vi "JTAG Commit.vi"(8 "error in (no error)":errorcluster) -> (0 "error out":errorcluster)   [LabVIEW 2010]
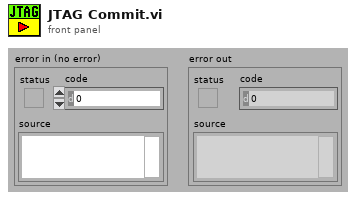
[diagram p1: front panel]
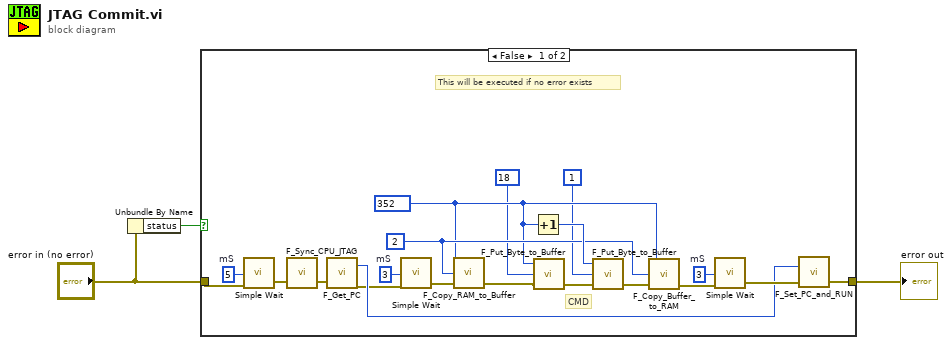
[diagram p0: block diagram]
diagram:
  n1 = Unbundle By Name("error in (no error)") -> ("status"=w2:bool)
  n2 = case shown="False" w2 {
    tunnel: [w10 w24] -> w3
    tunnel: "error in (no error)" -> [w4 w24]
    frame False {
      w6 = u32 5  # mS
      w19 = u32 3  # mS
      w20 = u32 3  # mS
      w16 = u16 2
      w9 = u16 352
      # "CMD"
      # "This will be executed if no error exists"
      n3 = call "Simple Wait.vi"("mS"=w6, "error in"=w4) -> ("error out"=w5:errorcluster)  [unwired: 12 in, 1 out]
      n4 = call "F_Sync_CPU_JTAG.vi"("error in (no error)"=w5) -> ("error out"=w13:errorcluster)  [unwired: 1 in, 1 out]
      n5 = call "F_Get_PC.vi"("error in (no error)"=w13) -> ("error out"=w11:errorcluster, "Program Counter"=w12:u16)  [unwired: 1 in]
      n6 = call "Simple Wait.vi"("mS"=w20, "error in"=w11) -> ("error out"=w17:errorcluster)  [unwired: 12 in, 1 out]
      n7 = call "F_Copy_RAM_to_Buffer.vi"("error in (no error)"=w17, "Block size to be copied"=w16, "RAM start address"=w9) -> ("error out"=w15:errorcluster)  [unwired: 2 in]
      n8 = Increment(x=w9) -> (x+1=w22:u16)
      n9 = call "F_Put_Byte_to_Buffer.vi"("error in (no error)"=w15, "New value"=u16 18, "Address of byte to be updated"=w9) -> ("error out"=w23:errorcluster)  [unwired: 2 in]
      n10 = call "F_Put_Byte_to_Buffer.vi"("error in (no error)"=w23, "New value"=u16 1, "Address of byte to be updated"=w22) -> ("error out"=w21:errorcluster)  [unwired: 2 in]
      n11 = call "F_Copy_Buffer_to_RAM.vi"("error in (no error)"=w21, "Block size to be copied"=w16, "Buffer start address"=w9) -> ("error out"=w18:errorcluster)  [unwired: 2 in]
      n12 = call "Simple Wait.vi"("mS"=w19, "error in"=w18) -> ("error out"=w14:errorcluster)  [unwired: 12 in, 1 out]
      n13 = call "F_Set_PC_and_RUN.vi"("error in (no error)"=w14, "PC start address"=w12) -> ("error out"=w10:errorcluster)  [unwired: 1 in]
    }
    frame True {
      # "Error exists, skip all functions"
    }
  }
  "error out" <- w3
